vi "Time Display.vi"(0 "RedPitaya connection in":refnum<k5>, 2 "Time Offset":dbl=-inf, 3 "Time Scale":dbl=-1.0, 5 "error in":errorcluster, 12 "timeout ms (2000)":i32=2000) -> (14 "RedPitaya connection out":refnum<k5>, 19 "error out":errorcluster)   [LabVIEW 2010, in "RedPitaya.lvlib"]
doc: "Sets time offset and scale"
uses:
  RedPitaya.lvlib
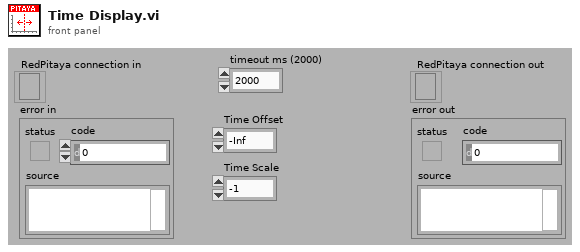
[diagram p1: front panel]
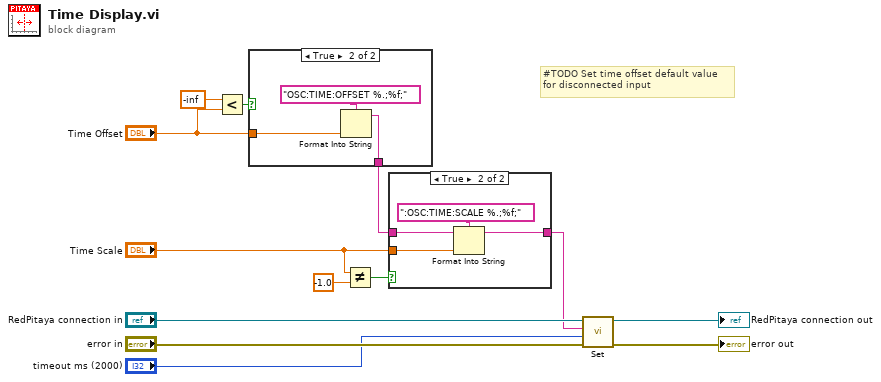
[diagram p0: block diagram]
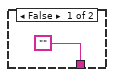
[diagram p3: hidden frame]
diagram:
  # "#TODO Set time offset default value\nfor disconnected input"
  n1 = Less?(x=-inf, y="Time Offset") -> (x < y?=w7:bool)
  n2 = case shown="True" w7 {
    tunnel: "Time Offset" -> [_ w15]
    tunnel: ["" w16] -> w9
    frame False {
    }
    frame True {
      n3 = Format Into String(format string="OSC:TIME:OFFSET %.;%f;", w15) -> (resulting string=w16:string)  [unwired: 2 in, 1 out]
    }
  }
  n4 = Not Equal?(x="Time Scale", y=-1.0) -> (x != y?=w4:bool)
  n5 = case shown="True" w4 {
    tunnel: w9 -> [w18 w22]
    tunnel: "Time Scale" -> [_ w19]
    tunnel: [w18 w20] -> w8
    frame False {
    }
    frame True {
      n6 = Format Into String(format string=":OSC:TIME:SCALE %.;%f;", initial string=w22, w19) -> (resulting string=w20:string)  [unwired: 1 in, 1 out]
    }
  }
  n7 = call "Set.vi"("error in"="error in", "timeout ms (2000)"="timeout ms (2000)", "SCPI Message"=w8, "RedPitaya connection in"="RedPitaya connection in") -> ("error out"=→"error out":errorcluster, "RedPitaya connection out"=→"RedPitaya connection out":refnum<k5>)  [unwired: 5 in, 1 out]
